vi "WLAN Tx Test Fetch DSSS Results.vi"(8 "error in (no error)":errorcluster, 11 "Template Tx Test in":refnum<class "niDTS WLAN Tx Test.lvclass">) -> (0 "error out":errorcluster, 2 "Results":T1 {"OBW"."Stop Frequency (Hz)" format="%#_4p"; "OBW"."Start Frequency (Hz)" format="%#_4p"; "OBW"."OBW (Hz)" format="%#_4p"}, 3 "Template Tx Test out":refnum<class "niDTS WLAN Tx Test.lvclass">)   [LabVIEW 2015, in "niDTS WLAN.lvlib" / "niDTS WLAN Tx Test.lvclass"]
uses:
  niDTS WLAN Tx Test.lvclass
  Includes/niDTS WLAN Tx Test INC DSSS Results.ctl
  Includes/niDTS WLAN Tx Test INC DSSS MOD EVM Results.ctl
  DSSS Tx Test/Includes/Results/niDTS WLAN DSSS Tx RES EVM ALL.ctl
  DSSS Tx Test/Includes/Results/niDTS WLAN DSSS Tx RES EVM RMS.ctl
  Includes/niDTS WLAN Tx Test INC TXP Results.ctl
  Includes/niDTS WLAN Tx Test INC TXP Result SINGLE.ctl
  Includes/niDTS WLAN Tx Test INC OBW Results.ctl
  Instrument/INSTR TX/Results/niDTS WLAN INSTR TX INC SEM Results.ctl
  Instrument/INSTR TX/Results/niDTS WLAN INSTR TX INC SEM FSEGemts Results.ctl
  Includes/Results/niDTS Tx RES INC SEM FSEGemts.ctl
  Instrument/INSTR TX/Results/niDTS WLAN INSTR TX INC SEM MARGin Results.ctl
  Includes/Results/niDTS Tx RES INC SEM Margin.ctl
  Includes/niDTS WLAN Tx Test INC DSSS MOD Impairments Results.ctl
  DSSS Tx Test/Includes/Results/niDTS WLAN DSSS Tx Impairmentsctl.ctl
  DSSS Tx Test/Includes/Results/niDTS WLAN DSSS Tx PowerRamp.ctl
  Instrument/INSTR TX/niDTS WLAN INSTR TX.lvclass
  Framework/Dut/Objects/BASE_class/niDTS Dut.lvclass
  niDTS WLAN.lvlib
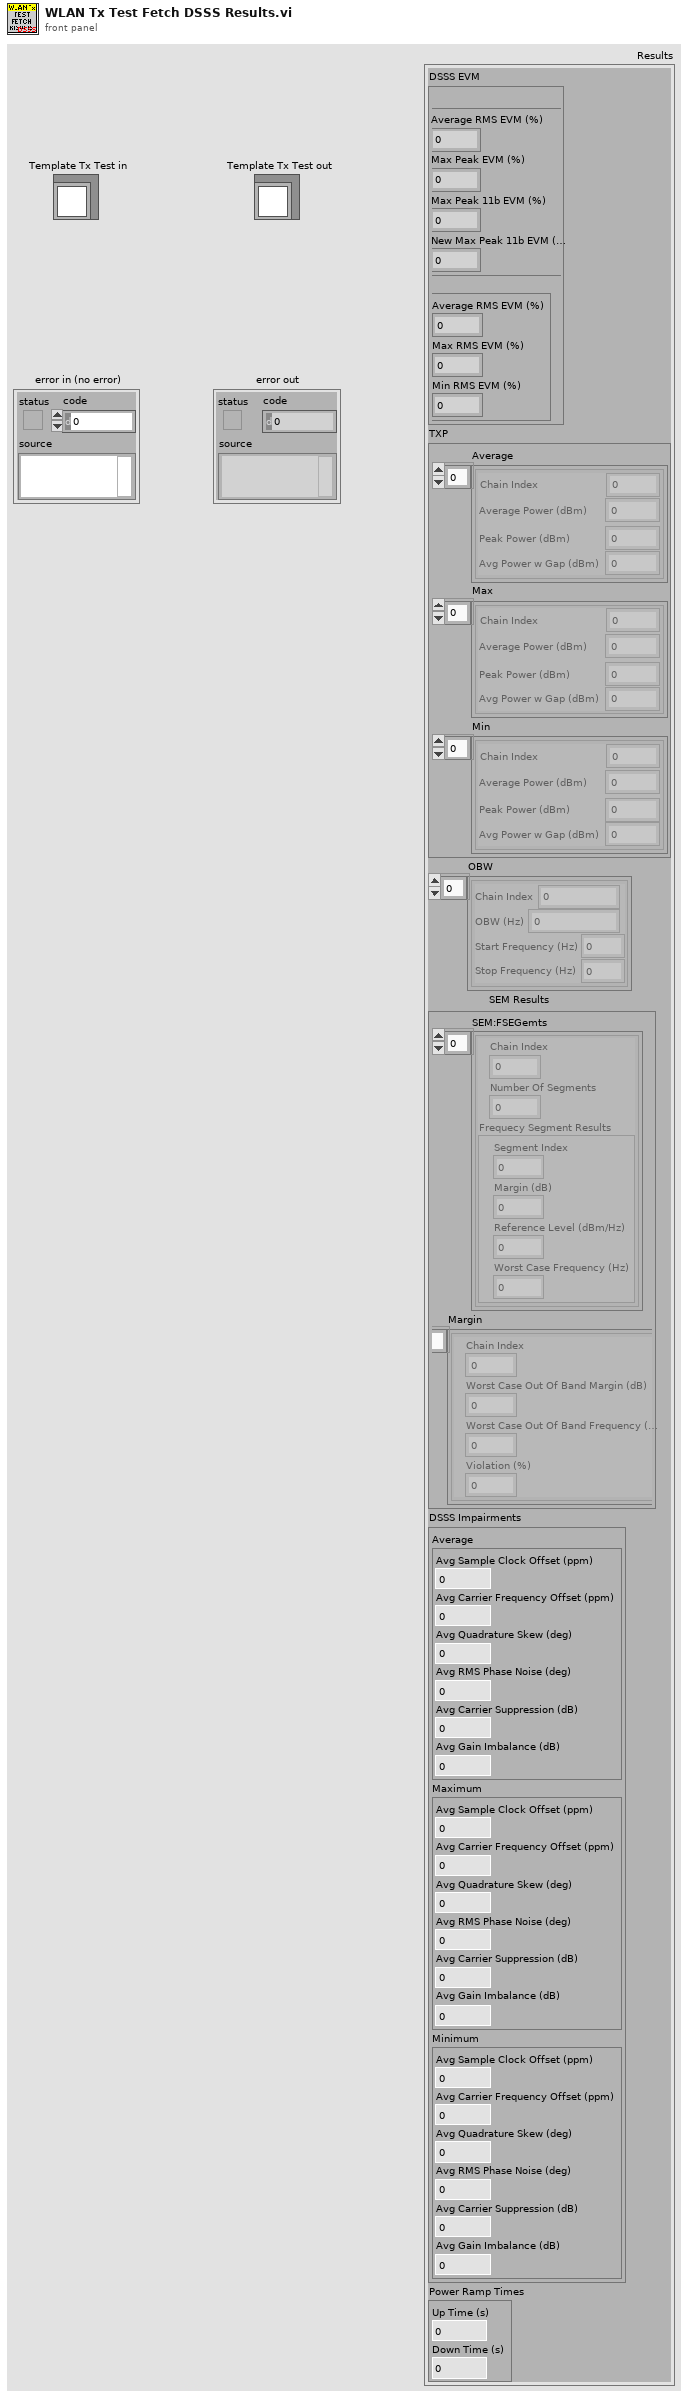
[diagram p1: front panel]
types:
  T1 = typedef "niDTS WLAN.lvlib/niDTS WLAN Tx Test INC DSSS Results.ctl" = cluster{"DSSS EVM":T2, "TXP":T5, "OBW":T7[], "SEM Results":T8, "DSSS Impairments":T13, "Power Ramp Times":T15}
  T2 = typedef "niDTS WLAN.lvlib/niDTS WLAN Tx Test INC DSSS MOD EVM Results.ctl" = cluster{"All":T3, "RMS":T4}
  T3 = typedef "niDTS WLAN.lvlib/niDTS WLAN DSSS Tx RES EVM ALL.ctl" = cluster{"Average RMS EVM (%)":dbl, "Max Peak EVM (%)":dbl, "Max Peak 11b EVM (%)":dbl, "New Max Peak 11b EVM (%)":dbl}
  T4 = typedef "niDTS WLAN.lvlib/niDTS WLAN DSSS Tx RES EVM RMS.ctl" = cluster{"Average RMS EVM (%)":dbl, "Max RMS EVM (%)":dbl, "Min RMS EVM (%)":dbl}
  T5 = typedef "niDTS WLAN.lvlib/niDTS WLAN Tx Test INC TXP Results.ctl" = cluster{"Average":T6[], "Max":T6[], "Min":T6[]}
  T6 = typedef "niDTS WLAN.lvlib/niDTS WLAN Tx Test INC TXP Result SINGLE.ctl" = cluster{"Chain Index":dbl, "Average Power (dBm)":dbl, "Peak Power (dBm)":dbl, "Avg Power w Gap (dBm)":dbl}
  T7 = typedef "niDTS WLAN.lvlib/niDTS WLAN Tx Test INC OBW Results.ctl" = cluster{"Chain Index":dbl, "OBW (Hz)":dbl, "Start Frequency (Hz)":dbl, "Stop Frequency (Hz)":dbl}
  T8 = typedef "niDTS WLAN.lvlib/niDTS WLAN INSTR TX.lvclass/niDTS WLAN INSTR TX INC SEM Results.ctl" = cluster{"SEM:FSEGemts":T9, "Margin":T11}
  T9 = typedef "niDTS WLAN.lvlib/niDTS WLAN INSTR TX.lvclass/niDTS WLAN INSTR TX INC SEM FSEGemts Results.ctl" = T10[]
  T10 = typedef "niDTS WLAN.lvlib/niDTS Tx RES INC SEM FSEGemts.ctl" = cluster{"Chain Index":i32, "Number Of Segments":i32, "Frequecy Segment Results":cluster{"Segment Index":i32, "Margin (dB)":dbl, "Reference Level (dBm/Hz)":dbl, "Worst Case Frequency (Hz)":dbl}}
  T11 = typedef "niDTS WLAN.lvlib/niDTS WLAN INSTR TX.lvclass/niDTS WLAN INSTR TX INC SEM MARGin Results.ctl" = T12[]
  T12 = typedef "niDTS WLAN.lvlib/niDTS Tx RES INC SEM Margin.ctl" = cluster{"Chain Index":i32, "Worst Case Out Of Band Margin (dB)":dbl, "Worst Case Out Of Band Frequency (Hz)":dbl, "Violation (%)":dbl}
  T13 = typedef "niDTS WLAN.lvlib/niDTS WLAN Tx Test INC DSSS MOD Impairments Results.ctl" = cluster{"Average":T14, "Maximum":T14, "Minimum":T14}
  T14 = typedef "niDTS WLAN.lvlib/niDTS WLAN DSSS Tx Impairmentsctl.ctl" = cluster{"Avg Sample Clock Offset (ppm)":dbl, "Avg Carrier Frequency Offset (ppm)":dbl, "Avg Quadrature Skew (deg)":dbl, "Avg RMS Phase Noise (deg)":dbl, "Avg Carrier Suppression (dB)":dbl, "Avg Gain Imbalance (dB)":dbl}
  T15 = typedef "niDTS WLAN.lvlib/niDTS WLAN DSSS Tx PowerRamp.ctl" = cluster{"Up Time (s)":dbl, "Down Time (s)":dbl}
  T16 = typedef "niDTS Framework.lvlib/niDTS Dut INC Handle.ctl" = refnum<data-value>
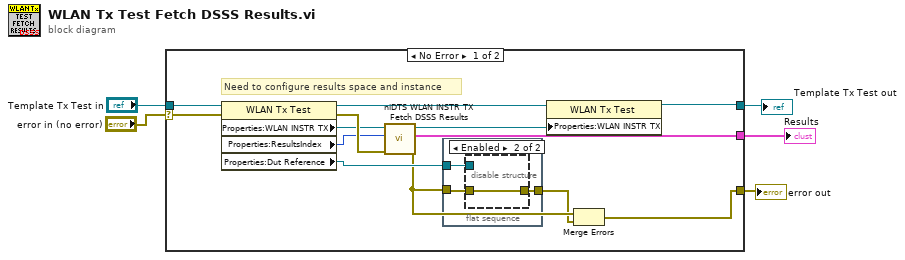
[diagram p0: block diagram]
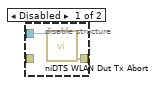
[diagram p2: hidden frame]
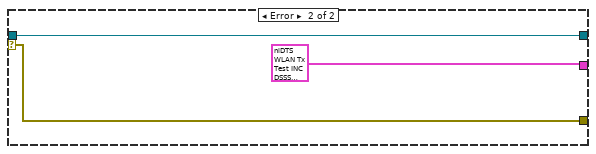
[diagram p3: hidden frame]
diagram:
  n1 = case shown="No Error" "error in (no error)" {
    selector: "error in (no error)" -> [w17 w27]
    tunnel: [w7 w27] -> w4
    tunnel: [w11 w26] -> w2
    tunnel: "Template Tx Test in" -> [w18 w26]
    tunnel: [w6 T1 {"DSSS EVM"={"All"={"Average RMS EVM (%)"=0.0, "Max Peak EVM (%)"=0.0, "Max Peak 11b EVM (%)"=0.0, "New Max Peak 11b EVM (%)"=0.0}, "RMS"={"Average RMS EVM (%)"=0.0, "Max RMS EVM (%)"=0.0, "Min RMS EVM (%)"=0.0}}, "TXP"={"Average"=[], "Max"=[], "Min"=[]}, "OBW"=[], "SEM Results"={"SEM:FSEGemts"=[], "Margin"=[]}, "DSSS Impairments"={"Average"={"Avg Sample Clock Offset (ppm)"=0.0, "Avg Carrier Frequency Offset (ppm)"=0.0, "Avg Quadrature Skew (deg)"=0.0, "Avg RMS Phase Noise (deg)"=0.0, "Avg Carrier Suppression (dB)"=0.0, "Avg Gain Imbalance (dB)"=0.0}, "Maximum"={"Avg Sample Clock Offset (ppm)"=0.0, "Avg Carrier Frequency Offset (ppm)"=0.0, "Avg Quadrature Skew (deg)"=0.0, "Avg RMS Phase Noise (deg)"=0.0, "Avg Carrier Suppression (dB)"=0.0, "Avg Gain Imbalance (dB)"=0.0}, "Minimum"={"Avg Sample Clock Offset (ppm)"=0.0, "Avg Carrier Frequency Offset (ppm)"=0.0, "Avg Quadrature Skew (deg)"=0.0, "Avg RMS Phase Noise (deg)"=0.0, "Avg Carrier Suppression (dB)"=0.0, "Avg Gain Imbalance (dB)"=0.0}}, "Power Ramp Times"={"Up Time (s)"=0.0, "Down Time (s)"=0.0}} ("DSSS Results")] -> w1
    frame No Error {
      # "Need to configure results space and instance"
      n2 = property class="WLAN Tx Test"(reference=w18, error in=w17) -> (reference out=w13:refnum<class "niDTS WLAN Tx Test.lvclass">, error out=w16:errorcluster, "Properties:WLAN INSTR TX"=w15:refnum<class "niDTS WLAN INSTR TX.lvclass">, "Properties:ResultsIndex"=w10:u8, "Properties:Dut Reference"=w14:T16)
      n3 = call-dynamic "niDTS WLAN INSTR TX Fetch DSSS Results.vi"("error in (no error)"=w16, "ActiveResultsSpace"=w10, "niDTS WLAN INSTR TX in"=w15) -> ("error out"=w9:errorcluster, "DSSS Results"=w6:T1, "niDTS WLAN INSTR TX out"=w12:refnum<class "niDTS WLAN INSTR TX.lvclass">)  [unwired: 6 in]
      n4 = flat-sequence {
        tunnel: w14 -> [w21]
        tunnel: [w20] -> w8
        tunnel: w9 -> [w19]
        frame #0 {
          n5 = disable-structure shown="Enabled" {
            disable-tunnel: w21 -> [w23 _]
            disable-tunnel: [w22 w24] -> w20
            disable-tunnel: w19 -> [_ w24]
            frame Disabled {
              n6 = call "niDTS WLAN Dut Tx Abort.vi"("WLAN Dut Handle in"=w23) -> ("error out"=w22:errorcluster)  [unwired: 13 in, 1 out]
            }
            frame Enabled {
            }
          }
        }
      }
      n7 = property class="WLAN Tx Test"(reference=w13, "Properties:WLAN INSTR TX"=w12) -> (reference out=w11:refnum<class "niDTS WLAN Tx Test.lvclass">)  [unwired: 1 in, 1 out]
      n8 = Merge Errors(w9, w8) -> (w7:errorcluster)
    }
    frame Error {
    }
  }
  "error out" <- w4
  "Template Tx Test out" <- w2
  "Results" <- w1
